vi "Wiimote Get Input Report.vi"(8 "error in":errorcluster, 10 "bInputReport":T1=48 items=["Status Information"=32, "Read Data"=33, "Write Data"=34, "Core Buttons"=48, "Core Buttons and Accelerometer"=49, "Core Buttons with 8 Extension bytes"=50, "Core Buttons and Accelerometer with 12 IR bytes"=51, "Core Buttons with 19 Extension bytes"=52, "Core Buttons and Accelerometer with 16 Extension Bytes"=53, "Core Buttons with 10 IR bytes and 9 Extension Bytes"=54, "Core Buttons and Accelerometer with 10 IR bytes and 6 Extension Bytes"=55], 11 "hWiimoteHandle in":u32 format="%08x") -> (0 "error out":errorcluster, 2 "pReportBuffer out":u8[](array[numeric]) format="%02x", 3 "hWiimoteHandle out":u32 format="%08x")   [LabVIEW 2010]
uses:
  Wiimote Reporting Mode.ctl
  C:/Windows/System32/hid.dll
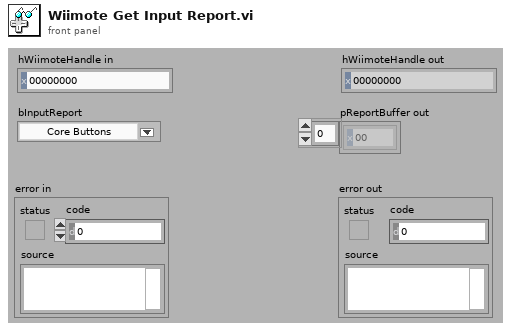
[diagram p1: front panel]
types:
  T1 = typedef "Wiimote Reporting Mode.ctl" = u8
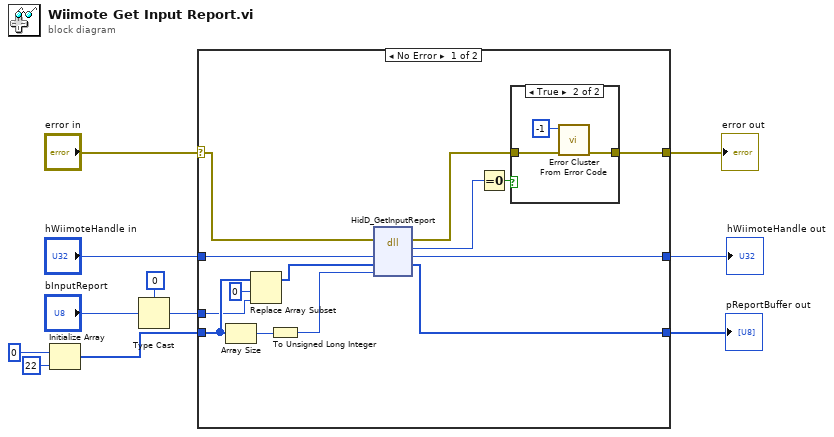
[diagram p0: block diagram]
diagram:
  n1 = Initialize Array(u8 0 ("element"), 22 ("dimension size")) -> (w4:u8[])
  n2 = Type Cast(type=u8 0 ("index"), x="bInputReport") -> (*(type *) &x=w1:u8)
  n3 = case shown="No Error" "error in" {
    selector: "error in" -> [w22 w32]
    tunnel: [w21 w32] -> w10
    tunnel: "hWiimoteHandle in" -> [w25 w31]
    tunnel: [w19 w31] -> w8
    tunnel: [w16 w30] -> w7
    tunnel: w4 -> [w15 w30]
    tunnel: w1 -> [w12 _]
    frame No Error {
      n4 = Array Size(array=w15) -> (size(s)=w24:i32)
      n5 = Replace Array Subset(array=w15, new element=w12, index=0) -> (w14:u8[])
      n6 = To Unsigned Long Integer(number=w24) -> (unsigned 32bit integer=w23:u32)
      n7 = dll-call lib="C:/Windows/System32/hid.dll" fn="HidD_GetInputReport"(error in=w22, "hWiimoteHandle"=w25, "pReportBuffer"=w14, "dwReportBufferLength"=w23) -> (error out=w20:errorcluster, "return type"=w17:u32, "hWiimoteHandle"=w19:u32, "pReportBuffer"=w16:u8[])  [unwired: 3 in, 1 out]
      n8 = Equal To 0?(x=w17) -> (x = 0?=w18:bool)
      n9 = case shown="True" w18 {
        tunnel: w20 -> [w26 w29]
        tunnel: [w26 w28] -> w21
        frame False {
        }
        frame True {
          n10 = call <vilib>:"Error Cluster From Error Code.vi"("error in (no error)"=w29, "error code (0)"=-1) -> ("error out"=w28:errorcluster)  [unwired: 7 in]
        }
      }
    }
    frame Error {
    }
  }
  "error out" <- w10
  "hWiimoteHandle out" <- w8
  "pReportBuffer out" <- w7
